vi "launcher.vi"   [LabVIEW 2023]
uses:
  <vilib>/ActorFramework/Actor/Actor.lvclass
  SLM_Controller.lvclass
  C:/Program Files/National Instruments/LabVIEW 2023/vi.lib/ActorFramework/Actor/Actor.lvclass
  C:/Users/quantum/Documents/LVDAQ/UIs/SLM_Controller/SLM_Controller/SLM_Controller/SLM_Controller.lvclass
  C:/Users/quantum/Documents/LVDAQ/Interfaces/InitDeinitInterface/InitDeinitComm/InitDeinitComm.lvclass
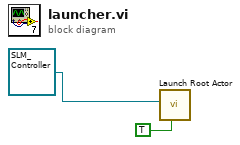
[diagram p0: block diagram]
diagram:
  n1 = call <vilib>:"Launch Root Actor.vi"("Open Actor Core front panel? (F)"=TRUE, "Actor"=refnum<class "SLM_Controller.lvclass"> refnum ("SLM_Controller.lvlib:SLM_Controller.lvclass")) -> ()  [unwired: 8 in, 2 out]
